vi "setLastPublishedTimeoutActuatorIds.vi"(10 "LastPublishedTimeoutActuatorIds":i32[](array[numeric]), 11 "Publisher in":refnum<class "Publisher.lvclass">) -> (3 "Publisher out":refnum<class "Publisher.lvclass">)   [LabVIEW 2016, in "Publisher.lvclass"]
uses:
  Publisher.lvclass
  Publisher.lvclass/Publisher.ctl
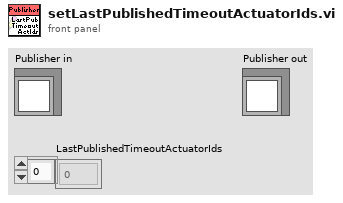
[diagram p1: front panel]
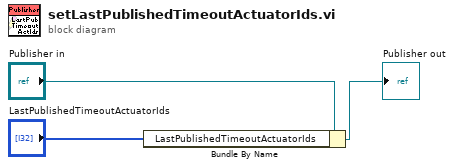
[diagram p0: block diagram]
diagram:
  n1 = Bundle By Name(cluster="Publisher in", "LastPublishedTimeoutActuatorIds"="LastPublishedTimeoutActuatorIds") -> (→"Publisher out":refnum<class "Publisher.lvclass">)
